vi "Array Transformations 2 LV2016 NIVerified.vi"() -> ()   [LabVIEW 2016]
panel:
  out "transpose":bool[][](array[boolean])
  out "rotate 270":bool[][](array[boolean])
  out "rotate 180":bool[][](array[boolean])
  out "rotate 90":bool[][](array[boolean])
  out "Diagonal flip":bool[][](array[boolean])
  out "Horizontal  flip":bool[][](array[boolean])
  out "Vertical flip":bool[][](array[boolean])
  in  "Input":bool[][](array[boolean])=[[FALSE, FALSE, TRUE, FALSE], [FALSE, TRUE, TRUE, FALSE], [FALSE, FALSE, TRUE, FALSE], [FALSE, FALSE, TRUE, FALSE], [TRUE, TRUE, TRUE, TRUE]]
  # "Overview:\nGiven a 2D array, there are 8 symmetry related transformations possible:\nidentity\nvertical flip\nhorizontal flip\nrotate 180 degrees\ntranspose\nrotate 90 degrees\nrotate 270 degrees\ndiagonal flip\nRequirements:\nLabVIEW 2012 (or compatible)\nInstructions:\nRun this VI"
  # "This VI shows how to apply all simple symmetry operations to a 2D array.\n\nChristian Altenbach, altenbach@gmail.com"
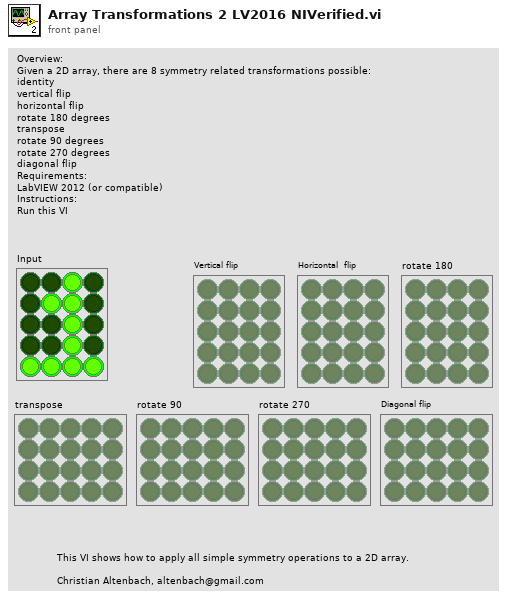
[diagram p1: front panel]
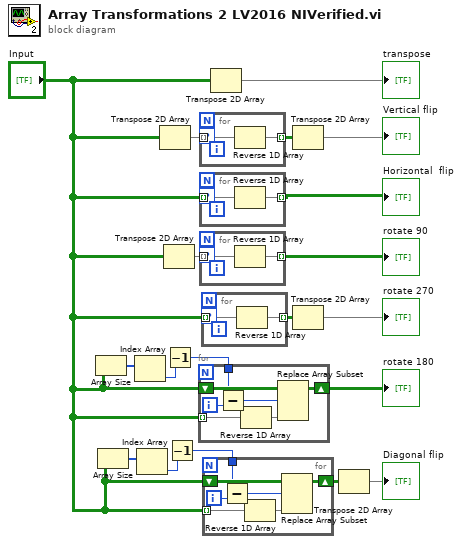
[diagram p0: block diagram]
diagram:
  n1 = Array Size(array="Input") -> (size(s)=w13:i32[])
  n2 = Array Size(array="Input") -> (size(s)=w8:i32[])
  n3 = Index Array(array=w13) -> (element=w11:i32)  [unwired: 1 in]
  n4 = Index Array(array=w8) -> (element=w10:i32)  [unwired: 1 in]
  n5 = Transpose 2D Array(2D array="Input") -> (transposed array=w2:bool[][])
  n6 = Transpose 2D Array(2D array="Input") -> (transposed array=w15:bool[][])
  n7 = Decrement(x=w11) -> (x-1=w12:i32)
  n8 = Decrement(x=w10) -> (x-1=w9:i32)
  n9 = for {
    shift-right: [w26] -> w14
    shift-left: "Input" -> [w25]
    tunnel: w12 -> [w23]
    tunnel: "Input" -> [w20] mode=indexing
    i -> [w24]
    n10 = Subtract(x=w23, y=w24) -> (x-y=w22:i32)
    n11 = Reverse 1D Array(array=w20) -> (reversed array=w21:bool[])
    n12 = Replace Array Subset(array=w25, new element=w21, index (row)=w22) -> (w26:bool[][])  [unwired: 1 in]
  }
  "rotate 180" <- w14
  n13 = for {
    tunnel: w2 -> [w28] mode=indexing
    tunnel: [w27] -> w3 mode=indexing
    workers-P: _ -> [_]
    n14 = Reverse 1D Array(array=w28) -> (reversed array=w27:bool[])
  }
  n15 = for {
    tunnel: "Input" -> [w30] mode=indexing
    tunnel: [w29] -> w5 mode=indexing
    workers-P: _ -> [_]
    n16 = Reverse 1D Array(array=w30) -> (reversed array=w29:bool[])
  }
  "Horizontal  flip" <- w5
  n17 = for {
    tunnel: w15 -> [w32] mode=indexing
    tunnel: [w31] -> w19 mode=indexing
    workers-P: _ -> [_]
    n18 = Reverse 1D Array(array=w32) -> (reversed array=w31:bool[])
  }
  "rotate 90" <- w19
  n19 = for {
    tunnel: "Input" -> [w34] mode=indexing
    tunnel: [w33] -> w18 mode=indexing
    workers-P: _ -> [_]
    n20 = Reverse 1D Array(array=w34) -> (reversed array=w33:bool[])
  }
  n21 = for {
    shift-right: [w41] -> w7
    shift-left: "Input" -> [w40]
    tunnel: w9 -> [w38]
    tunnel: "Input" -> [w35] mode=indexing
    i -> [w39]
    n22 = Subtract(x=w38, y=w39) -> (x-y=w37:i32)
    n23 = Reverse 1D Array(array=w35) -> (reversed array=w36:bool[])
    n24 = Replace Array Subset(array=w40, new element=w36, index (row)=w37) -> (w41:bool[][])  [unwired: 1 in]
  }
  n25 = Transpose 2D Array(2D array="Input") -> (transposed array=→"transpose":bool[][])
  n26 = Transpose 2D Array(2D array=w3) -> (transposed array=→"Vertical flip":bool[][])
  n27 = Transpose 2D Array(2D array=w18) -> (transposed array=→"rotate 270":bool[][])
  n28 = Transpose 2D Array(2D array=w7) -> (transposed array=→"Diagonal flip":bool[][])
